vi "Pre Loop Init.vi"(8 "error in":errorcluster, 10 "Ref In":refnum<vi>) -> (0 "error out":errorcluster, 3 "Event Registration Refnum":refnum<event-registration>)   [LabVIEW 2018, in "Sensor Interface.lvlib"]
uses:
  Sensor Interface.lvlib
  Private Controls/Module Data Cluster.ctl
  Private Controls/Module Action.ctl
  User Events/controls/Actions.ctl
  Private Controls/Queue FG Action.ctl
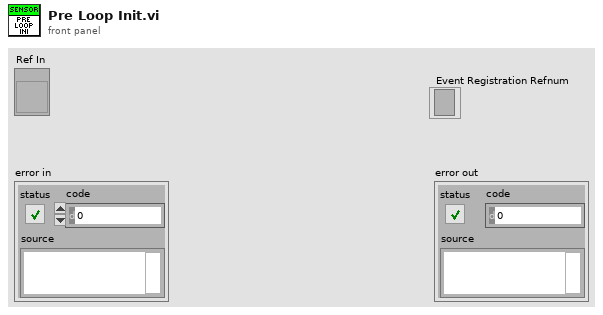
[diagram p1: front panel]
types:
  T1 = typedef "Sensor Interface.lvlib/Queue FG Action.ctl" = enum16{"Release", "Get", "Set"}
  T2 = typedef "Actions.ctl" = enum16{"Get", "Create", "Destroy"}
  T3 = typedef "Sensor Interface.lvlib/Module Data Cluster.ctl" = cluster{"Variant":variant, "action":T4}
  T4 = typedef "Sensor Interface.lvlib/Module Action.ctl" = enum16{"error", "exit", "init", "Start Sim", "Update Position"}
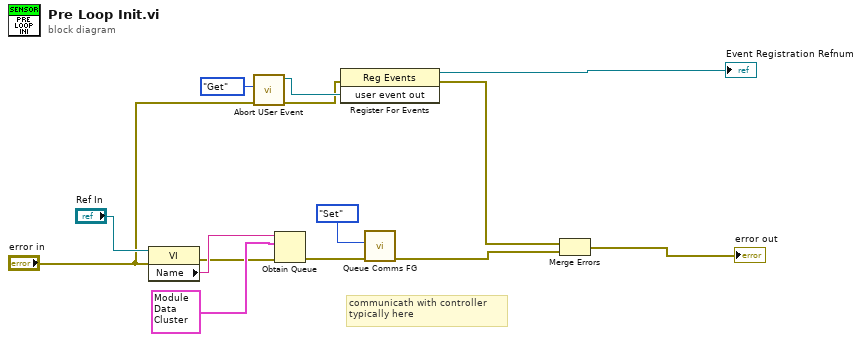
[diagram p0: block diagram]
diagram:
  # "communicath with controller typically here"
  n1 = property class="VI"(reference="Ref In", error in="error in") -> (error out=w9:errorcluster, "Name"=w13:string)  [unwired: 1 out]
  n2 = call "Abort USer Event.vi"("error in"="error in", "Enum"=Actions."Get") -> ("error out"=w3:errorcluster, "user event out"=w6:refnum<user-event>)  [unwired: 8 in]
  n3 = Obtain Queue(name (unnamed)=w13, element data type=T3 {"Variant"=variant, "action"=enum."init"} ("Module Data Cluster"), error in (no error)=w9) -> (error out=w11:errorcluster)  [unwired: 2 in, 2 out]
  n4 = register-events(error in=w3, w6) -> (reference out=→"Event Registration Refnum":refnum<event-registration>, error out=w5:errorcluster)  [unwired: 1 in]
  n5 = call "Queue Comms FG.vi"("error in"=w11, "Action"=Queue_FG_Action."Set") -> ("error out"=w1:errorcluster)  [unwired: 8 in, 1 out]
  n6 = Merge Errors(w5, w1) -> (→"error out":errorcluster)
